vi "Write VISA Address.vi"(8 "error in (no error)":errorcluster, 10 "VISA Address":refnum<visa-resource-name>, 11 "Lutron QS Object in":refnum<class "Lutron QS Object.lvclass">) -> (0 "error out":errorcluster, 3 "Lutron QS Object out":refnum<class "Lutron QS Object.lvclass">)   [LabVIEW 2014]
uses:
  Lutron QS Object.lvclass
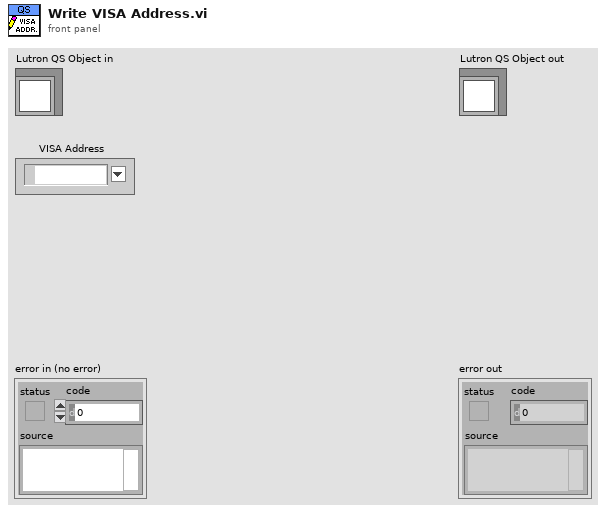
[diagram p1: front panel]
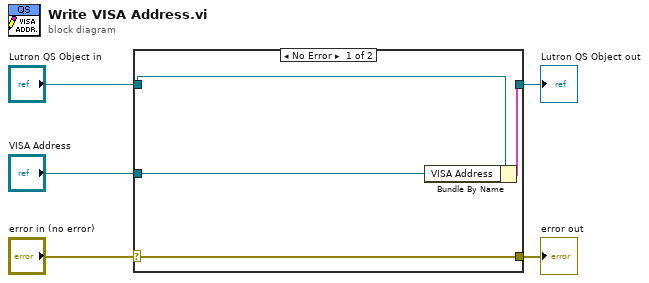
[diagram p0: block diagram]
diagram:
  n1 = case shown="No Error" "error in (no error)" {
    selector: "error in (no error)" -> [w9 w10]
    tunnel: [w9 w10] -> w4
    tunnel: [w7 w11] -> w2
    tunnel: "Lutron QS Object in" -> [w8 w11]
    tunnel: "VISA Address" -> [w6 _]
    frame No Error {
      n2 = Bundle By Name(cluster=w8, "VISA Address"=w6) -> (w7:cluster{})
    }
    frame Error {
    }
  }
  "error out" <- w4
  "Lutron QS Object out" <- w2
